vi "_Get Cell.vi"(8 "error in":errorcluster, 10 "Cell Address":string, 11 "Row in":refnum<k24>) -> (0 "error out":errorcluster, 2 "Cell":refnum<k24>, 3 "Row out":refnum<k24>)   [LabVIEW 2021, in "Open Xml.lvlib"]
uses:
  Open Xml.lvlib
  D:/git/Open-Xml-LabVIEW/dll/DocumentFormat.OpenXml.dll
  dll/DocumentFormat.OpenXml.dll
  D:/git/Open-Xml-LabVIEW/dll/DocumentFormat.OpenXml.Framework.dll
  dll/DocumentFormat.OpenXml.Framework.dll
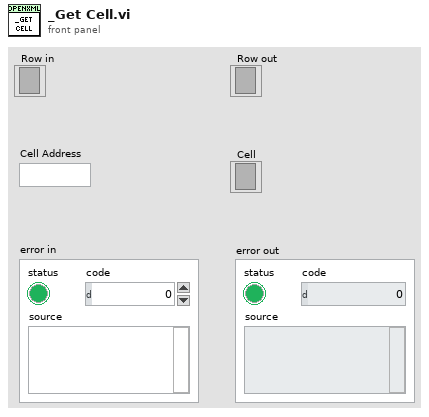
[diagram p1: front panel]
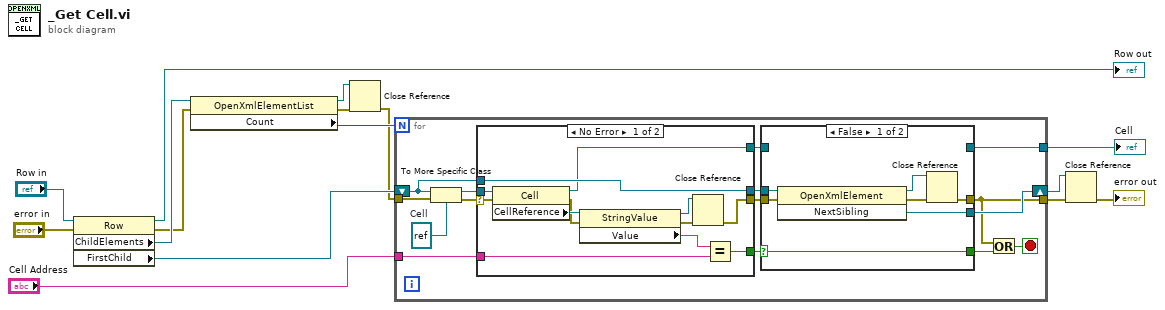
[diagram p0: block diagram]
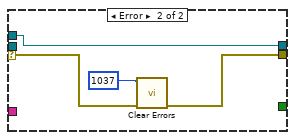
[diagram p3: hidden frame]
diagram:
  n1 = property class="Row"(reference="Row in", error in="error in") -> (reference out=→"Row out":refnum<k24>, error out=w7:errorcluster, "ChildElements"=w15:refnum<k24>, "FirstChild"=w13:refnum<k24>)
  n2 = property class="OpenXmlElementList"(reference=w15, error in=w7) -> (reference out=w10:refnum<k24>, error out=w9:errorcluster, "Count"=w14:i32)
  n3 = Close Reference(reference=w10, error in (no error)=w9) -> (error out=w8:errorcluster)
  n4 = for {
    N: w14 -> [_]
    tunnel: w8 -> [w29]
    tunnel: [w20] -> w12
    shift-right: [w21] -> w11
    shift-left: w13 -> [w27]
    tunnel: "Cell Address" -> [w25]
    tunnel: [w16] -> w1
    stop <- w24 stop-if-true
    w30 = refnum<k24> refnum  # Cell
    n5 = To More Specific Class(target class=w30, reference=w27, error in=w29) -> (specific class reference=w26:refnum<k24>, error out=w28:errorcluster)
    n6 = case shown="No Error" w28 {
      selector: w28 -> [w52 w56]
      tunnel: [w41 w54] -> w23
      tunnel: w27 -> [w46 w55]
      tunnel: [w46 w55] -> w22
      tunnel: [w47 _] -> w19
      tunnel: w26 -> [w51 _]
      tunnel: w25 -> [w48 _]
      tunnel: [w45 _] -> w17
      frame No Error {
        n7 = property class="Cell"(reference=w51, error in=w52) -> (reference out=w45:refnum<k24>, error out=w44:errorcluster, "CellReference"=w50:refnum<k24>)
        n8 = property class="StringValue"(reference=w50, error in=w44) -> (reference out=w42:refnum<k24>, error out=w43:errorcluster, "Value"=w49:string)
        n9 = Close Reference(reference=w42, error in (no error)=w43) -> (error out=w41:errorcluster)
        n10 = Equal?(x=w49, y=w48) -> (x = y?=w47:bool)
      }
      frame Error {
        n11 = call <vilib>:"Clear Errors.vi"("error in (no error)"=w56, "specific error code to clear (0: all)"=1037) -> ("error out"=w54:errorcluster)  [unwired: 4 in, 1 out]
      }
    }
    n12 = case shown="False" w19 {
      selector: w19 -> [w31 w40]
      tunnel: w23 -> [w37 w39]
      tunnel: w22 -> [w35 _]
      tunnel: [w34 _] -> w21
      tunnel: [w32 w39] -> w20
      tunnel: [w31 w40] -> w18
      tunnel: w17 -> [_ w38]
      tunnel: [_ w38] -> w16
      frame False {
        n13 = invoke class="OpenXmlElement" method="NextSibling"(reference=w35, error in=w37) -> (reference out=w33:refnum<k24>, error out=w36:errorcluster, "NextSibling"=w34:refnum<k24>)  [unwired: 1 in]
        n14 = Close Reference(reference=w33, error in (no error)=w36) -> (error out=w32:errorcluster)
      }
      frame True {
      }
    }
    n15 = Or(x=w20, y=w18) -> (x .or. y?=w24:bool)
  }
  "Cell" <- w1
  n16 = Close Reference(reference=w11, error in (no error)=w12) -> (error out=→"error out":errorcluster)
